vi "GTH_V2.String2CalibrationData.vi"(8 "错误输入":errorcluster, 11 "String":string) -> (0 "错误输出":errorcluster, 1 "Para":dbl[](array[numeric]), 2 "Count":u32, 3 "OK?":bool, 4 "Date":T1 caption="输出簇", 5 "Code":string)   [LabVIEW 2012, in "Lib_UEL.ATE.lvlib" / "STM32-CoreBD.lvlib"]
uses:
  STM32-CoreBD.lvlib
  <vilib>/Utility/miscctls.llb/LVDateTimeRec.ctl
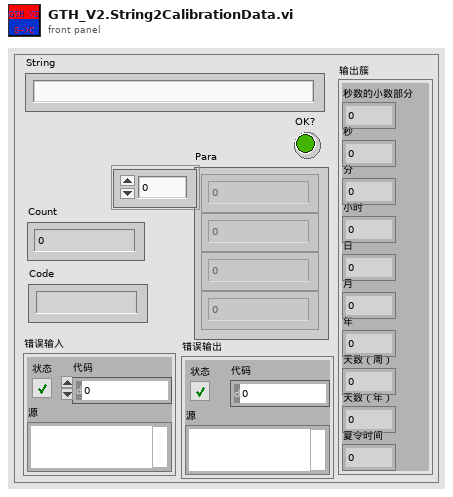
[diagram p1: front panel]
types:
  T1 = typedef "LVDateTimeRec.ctl" = cluster{"fractional second":dbl, "second":i32, "minute":i32, "hour":i32, "day of month":i32, "month":i32, "year":i32, "day of week":i32, "day of year":i32, "DST":i32}
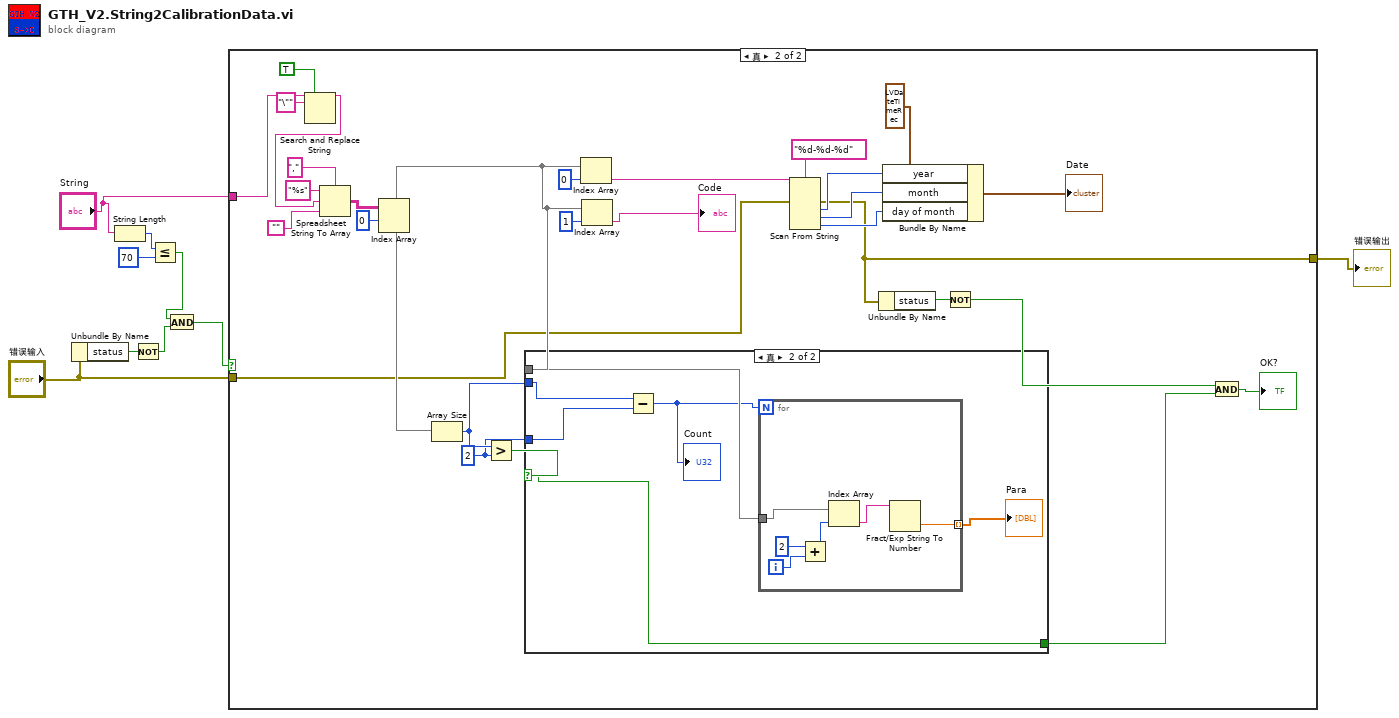
[diagram p0: block diagram]
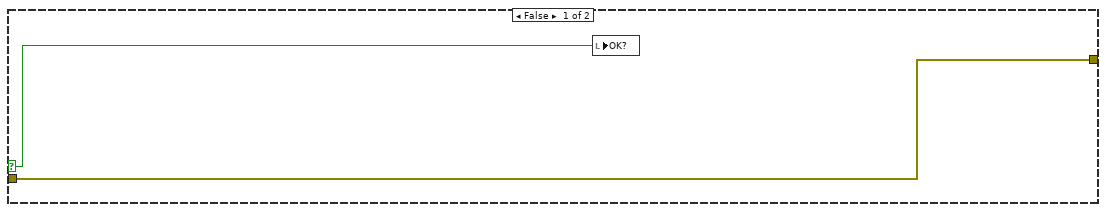
[diagram p2: hidden frame]
diagram:
  n1 = Unbundle By Name("错误输入") -> ("status"=w4:bool)
  n2 = String Length(string="String") -> (length=w7:i32)
  n3 = Not(x=w4) -> (.not. x?=w3:bool)
  n4 = Less Or Equal?(x=w7, y=70) -> (x <= y?=w5:bool)
  n5 = And(x=w5, y=w3) -> (x .and. y?=w2:bool)
  n6 = case shown="真" w2 {
    selector: w2 -> [w10 _]
    tunnel: [w11 w17] -> w9
    tunnel: "String" -> [_ w13]
    tunnel: "错误输入" -> [w11 w16]
    frame False {
      n7 = local write "OK?"(w10) -> ()
    }
    frame True {
      w31 = 2 ("y")
      n8 = Search and Replace String(replace all?=TRUE ("替换全部？(F)"), input string=w13, search string="\"" ("搜索字符串")) -> (result string=w12:string)  [unwired: 5 in, 3 out]
      n9 = Spreadsheet String To Array(delimiter (Tab)="," ("分隔符(Tab)"), format string="%s" ("格式字符串"), spreadsheet string=w12, array type (2D Dbl)="") -> (array=w37:string[][])
      n10 = Index Array(array=w37, index (row)=0 ("索引 (行)")) -> (element=w30:string[])  [unwired: 1 in]
      n11 = Array Size(array=w30) -> (size(s)=w32:i32)
      n12 = Greater?(x=w32, y=w31) -> (0:w33:bool)
      n13 = case shown="真" w33 {
        selector: w33 -> [w41 w42]
        tunnel: w32 -> [_ w47]
        tunnel: w31 -> [_ w46]
        tunnel: w30 -> [_ w45]
        tunnel: [w41 w42] -> w21
        frame False {
        }
        frame True {
          n14 = Subtract(x=w47, y=w46) -> (x-y=w44:i32)
          "Count" <- w44
          n15 = for {
            N: w44 -> [_]
            tunnel: w45 -> [w51]
            tunnel: [w48] -> w43 mode=indexing
            i -> [w53]
            n16 = Add(x=2, y=w53) -> (x+y=w50:i32)
            n17 = Index Array(array=w51, index=w50) -> (element=w49:string)
            n18 = Fract/Exp String To Number(string=w49) -> (number=w48:dbl)  [unwired: 3 in, 1 out]
          }
          "Para" <- w43
        }
      }
      n19 = Index Array(array=w30, index=0 ("索引")) -> (element=w29:string)
      n20 = Index Array(array=w30, index=1 ("索引")) -> (element=→"Code":string)
      n21 = Scan From String(format string="%d-%d-%d" ("格式字符串"), input string=w29, error in=w16) -> (error out=w17:errorcluster, output 1=w26:i32, output 2=w25:i32, output 3=w24:i32)  [unwired: 4 in, 2 out]
      n22 = Unbundle By Name(w17) -> ("status"=w20:bool)
      n23 = Bundle By Name(cluster=T1 {"fractional second"=0.0, "second"=0, "minute"=0, "hour"=0, "day of month"=0, "month"=0, "year"=0, "day of week"=0, "day of year"=0, "DST"=0} ("日期时间记录"), "year"=w26, "month"=w25, "day of month"=w24) -> (→"Date":T1)
      n24 = Not(x=w20) -> (.not. x?=w19:bool)
      n25 = And(x=w19, y=w21) -> (x .and. y?=→"OK?":bool)
    }
  }
  "错误输出" <- w9
